vi "Publish Sample.vi"(8 "error in (no error)":errorcluster, 9 "Sample":refnum<class "Sample.lvclass">, 10 "Sample Line (All Closed)":T1, 11 "Sample Line in":refnum<class "Sample Line.lvclass">) -> (0 "error out":errorcluster, 3 "Sample Line in 2":refnum<class "Sample Line.lvclass">)   [LabVIEW 2015, in "cRIO-Carbondioxide.lvlib" / "CO2-Actor.lvlib" / "Sample Line.lvclass"]
uses:
  Sample Line.lvclass
  Controls/Sample Line State Enumerator.ctl
  subs/Sample/Sample.lvclass
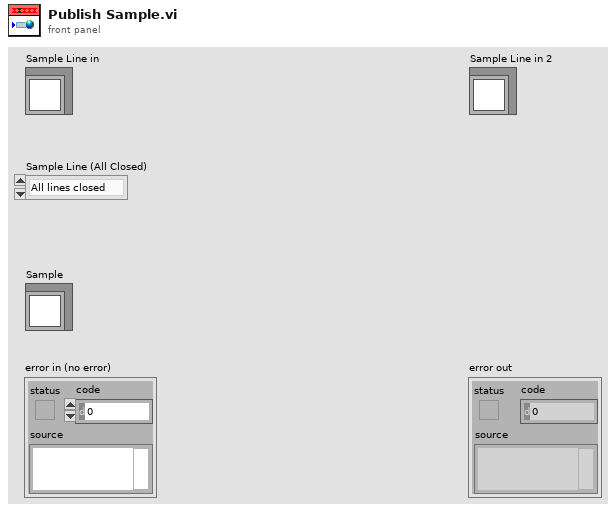
[diagram p1: front panel]
types:
  T1 = typedef "Sample Line State Enumerator.ctl" = enum16{"All lines closed", "Sample line 1.", "Sample line 2.", "Sample line 3.", "Sample line 4.", "Sample line 5.", "Out of range"}
  T2 = typedef "Sample Container.ctl" = cluster{"Sample In":refnum<k21>, "Sample Name":refnum<k21>, "Ti Cathode":refnum<k21>, "SampleQ":refnum<queue>}
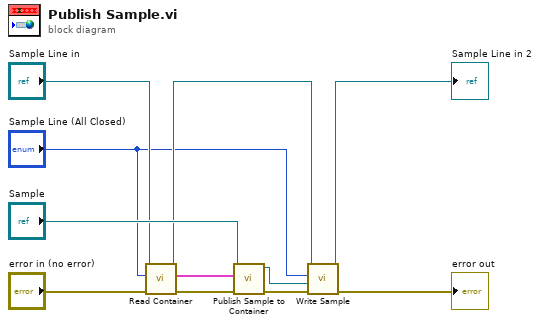
[diagram p0: block diagram]
diagram:
  n1 = call "Read Container.vi"("error in (no error)"="error in (no error)", "Sample Line (All Closed)"="Sample Line (All Closed)", "Sample Line in"="Sample Line in") -> ("error out"=w9:errorcluster, "Containers"=w1:T2[], "Sample Line out"=w5:refnum<class "Sample Line.lvclass">)  [unwired: 5 in, 1 out]
  n2 = call "Publish Sample to Container.vi"("error in (no error)"=w9, "Containers"=w1, "Sample in"="Sample") -> ("error out"=w7:errorcluster, "Sample out"=w3:refnum<class "Sample.lvclass">)  [unwired: 7 in]
  n3 = call "Write Sample.vi"("error in (no error)"=w7, "Sample 2"=w3, "Sample Line (All Closed)"="Sample Line (All Closed)", "Sample Line in"=w5) -> ("error out"=→"error out":errorcluster, "Sample Line out"=→"Sample Line in 2":refnum<class "Sample Line.lvclass">)  [unwired: 6 in]
